vi "Q8381 CURSOR DATA.vi"(1 "mode":u16(ring) items=["NORMAL", "delta MODE", "2ND  PEAK", "POWER", "P-P"], 2 "GPIB Address":u16=8 max=31 step=1, 3 "VISA resource name":refnum<visa-resource-name>) -> (0 "GPIB Status":bool)   [LabVIEW 2017]
doc: "mode:\n 0: Normal, 1: delta mode,\n 2: 2ND Peak, 3: Power,\n 4: P-P."
panel:
  out "Program Code":string
  # "CURSOR  DATA"
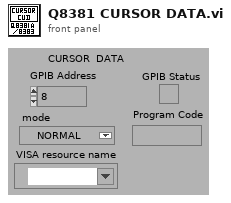
[diagram p1: front panel]
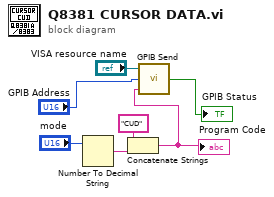
[diagram p0: block diagram]
diagram:
  n1 = Number To Decimal String(number="mode") -> (decimal integer string=w7:string)  [unwired: 1 in]
  n2 = Concatenate Strings("CUD", w7) -> (w1:string)
  "Program Code" <- w1
  n3 = call "GPIB Send.vi"("Command String"=w1, "Address"="GPIB Address", "VISA resource name"="VISA resource name") -> ("Error"=→"GPIB Status":bool)
